vi "Send Settings.vi"(8 "error in (no error)":errorcluster, 11 "N5745A in":refnum<class "5745A.lvclass">) -> (0 "error out":errorcluster, 3 "N5745A out":refnum<class "5745A.lvclass">)   [LabVIEW 2018, in "5745A.lvlib" / "5745A.lvclass"]
doc: "This Override method sends voltage, current and output settings to N5745A Power Supply. Voltage and Current are verified that they do not exceed the instrument's rating."
uses:
  5745A.lvclass
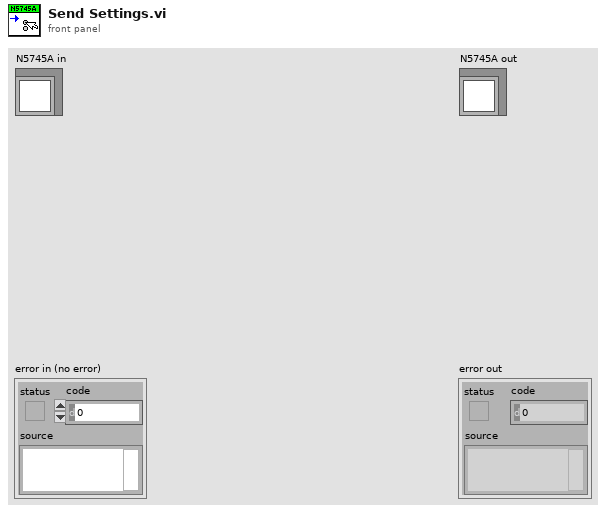
[diagram p1: front panel]
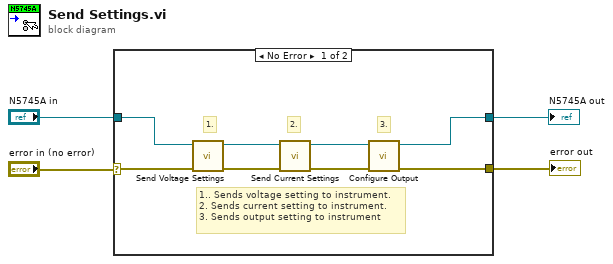
[diagram p0: block diagram]
diagram:
  n1 = case shown="No Error" "error in (no error)" {
    selector: "error in (no error)" -> [w5 w13]
    tunnel: "N5745A in" -> [w6 w14]
    tunnel: [w8 w14] -> w3
    tunnel: [w7 w13] -> w2
    frame No Error {
      # "1.. Sends voltage setting to instrument.\n2. Sends current setting to instrument.\n3. Sends output setting to instrument"
      # "3."
      # "2."
      # "1."
      n2 = call "Send Voltage Settings.vi"("error in (no error)"=w5, "N5745A in"=w6) -> ("error out"=w11:errorcluster, "N5745A out"=w12:refnum<class "5745A.lvclass">)  [unwired: 8 in]
      n3 = call "Send Current Settings.vi"("error in (no error)"=w11, "N5745A in"=w12) -> ("error out"=w10:errorcluster, "N5745A out"=w9:refnum<class "5745A.lvclass">)  [unwired: 8 in]
      n4 = call "Configure Output.vi"("error in (no error)"=w10, "N5745A in"=w9) -> ("error out"=w7:errorcluster, "N5745A out"=w8:refnum<class "5745A.lvclass">)  [unwired: 8 in]
    }
    frame Error {
    }
  }
  "error out" <- w2
  "N5745A out" <- w3
